vi "AFM_Driver_Manager.Abort.vi"(6 "Force? (F)":bool, 8 "error in (no error)":errorcluster, 11 "AFM_Driver_Manager in":refnum<class "AFM_Driver_Manager.lvclass">) -> (0 "error out":errorcluster, 3 "AFM_Driver_Manager out":refnum<class "AFM_Driver_Manager.lvclass">)   [LabVIEW 2019, in "AFM_Driver_Manager.lvclass"]
uses:
  AFM_Driver_Manager.lvclass
  AFM_Driver_Manager.lvclass/AFM_Driver_Manager.ctl
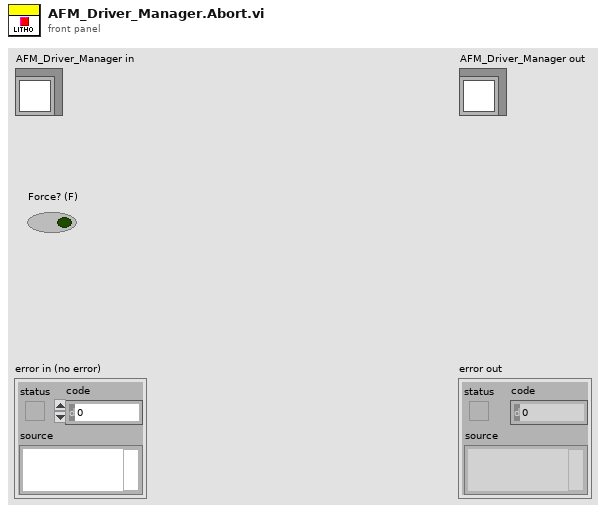
[diagram p1: front panel]
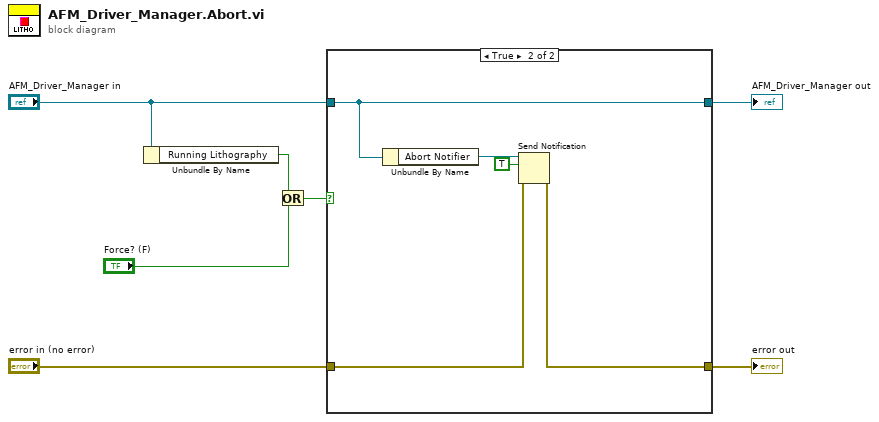
[diagram p0: block diagram]
diagram:
  n1 = Unbundle By Name("AFM_Driver_Manager in") -> ("Running Lithography"=w1:bool)
  n2 = Or(x=w1, y="Force? (F)") -> (x .or. y?=w2:bool)
  n3 = case shown="True" w2 {
    tunnel: "AFM_Driver_Manager in" -> [w9 w14]
    tunnel: [w9 w14] -> w6
    tunnel: [w8 w11] -> w5
    tunnel: "error in (no error)" -> [w8 w10]
    frame False {
    }
    frame True {
      n4 = Unbundle By Name(w14) -> ("Abort Notifier"=w13:refnum<notifier>)
      n5 = Send Notification(notification=TRUE, notifier=w13, error in (no error)=w10) -> (error out=w11:errorcluster)  [unwired: 1 out]
    }
  }
  "error out" <- w5
  "AFM_Driver_Manager out" <- w6
